vi "F Dwf Analog Out Limitation Info.vi"(7 "pMax":dbl, 8 "error in (no error)":errorcluster, 9 "pMin":dbl, 10 "idxChannel":i32, 11 "hdwf":i32) -> (0 "error out":errorcluster, 1 "pMin out":dbl, 3 "function return":i32, 5 "pMax out":dbl)   [LabVIEW 2019, in "Olasdwf.lvlib"]
doc: "DWFAPI int FDwfAnalogOutLimitationInfo(HDWF hdwf, int idxChannel, double *pMin, double *pMax);"
uses:
  Olasdwf.lvlib
  Windows/System32/dwf.dll
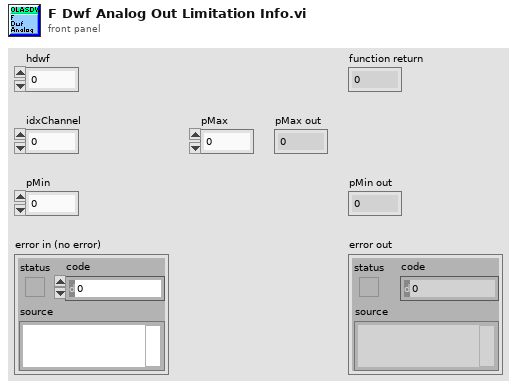
[diagram p1: front panel]
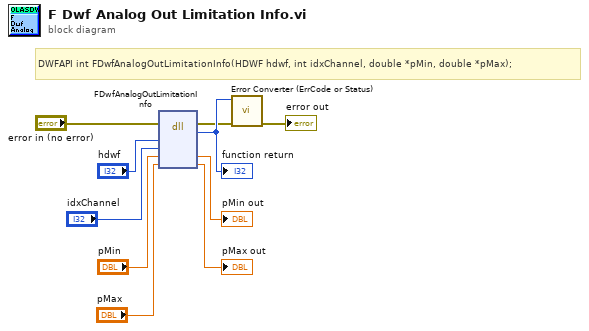
[diagram p0: block diagram]
diagram:
  # "DWFAPI int FDwfAnalogOutLimitationInfo(HDWF hdwf, int idxChannel, double *pMin, double *pMax);"
  n1 = dll-call lib="C:/Windows/System32/dwf.*" fn="FDwfAnalogOutLimitationInfo"(error in="error in (no error)", "hdwf"="hdwf", "idxChannel"="idxChannel", "pMin"="pMin", "pMax"="pMax") -> (error out=w2:errorcluster, w10:i32, "pMin"=→"pMin out":dbl, "pMax"=→"pMax out":dbl)  [unwired: 4 in, 1 out]
  "function return" <- w10
  n2 = call "Error Converter (ErrCode or Status).vi"("error in (no error)"=w2, "error code"=w10) -> ("error out"=→"error out":errorcluster)  [unwired: 9 in]
